vi "Lift Encoder test.vi"() -> ()   [LabVIEW 2014]
panel:
  in  "Reset Encoder?":bool
  in  "stop":bool
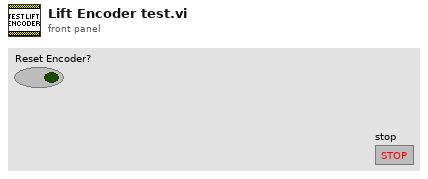
[diagram p1: front panel]
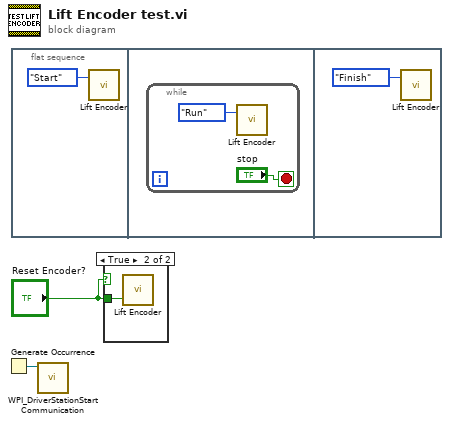
[diagram p0: block diagram]
diagram:
  n1 = Generate Occurrence() -> (w2:refnum<k4>)
  n2 = flat-sequence {
    frame #0 {
      n3 = call "Lift Encoder.vi"("Mode"=enum8{"Start", "Run", "Finish"}."Start") -> ()  [unwired: 1 in, 1 out]
    }
    frame #1 {
      n4 = while {
        stop <- "stop" stop-if-true
        n5 = call "Lift Encoder.vi"("Mode"=enum8{"Start", "Run", "Finish"}."Run") -> ()  [unwired: 1 in, 1 out]
      }
    }
    frame #2 {
      n6 = call "Lift Encoder.vi"("Mode"=enum8{"Start", "Run", "Finish"}."Finish") -> ()  [unwired: 1 in, 1 out]
    }
  }
  n7 = call <vilib>:"WPI_DriverStationStart Communication.vi"("occurrence"=w2) -> ()  [unwired: 11 in]
  n8 = case shown="True" "Reset Encoder?" {
    tunnel: "Reset Encoder?" -> [_ w7]
    frame False {
    }
    frame True {
      n9 = call "Lift Encoder.vi"("Reset"=w7) -> ()  [unwired: 1 in, 1 out]
    }
  }
